vi "timing_channel_reference.get.vi"(8 "error in (no error)":errorcluster, 11 "Item Ref in":T1 format="%.0x") -> (0 "error out":errorcluster, 2 "Timing Channel Ref":T1=18446744073709551615 format="%.0x", 3 "Item Ref out":T1=18446744073709551615 format="%.0x")   [LabVIEW 2024, in "Nominal Client Scripting.lvlib"]
uses:
  <vilib>/NI VeriStand/Custom Device API/Custom Device Item Ref.ctl
  Nominal Client Scripting.lvlib
  <vilib>/NI VeriStand/Custom Device Tools/Custom Device Utility Library/Custom Device Utility Library.lvlib
  <vilib>/NI VeriStand/Custom Device API/Custom Device API.lvlib
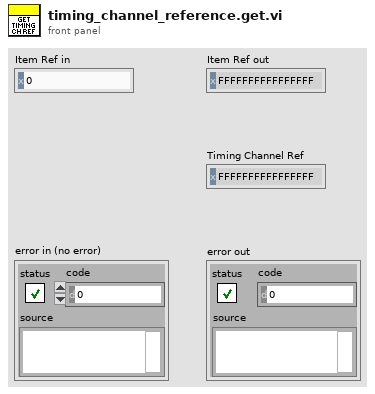
[diagram p1: front panel]
types:
  T1 = typedef "Custom Device API.lvlib/Custom Device Item Ref.ctl" = u64
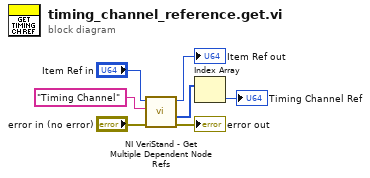
[diagram p0: block diagram]
diagram:
  n1 = call <vilib>:"NI VeriStand - Get Multiple Dependent Node Refs.vi"("error in (no error)"="error in (no error)", "Base Property Name"="Timing Channel" ("Property Name"), "Item Ref in"="Item Ref in") -> ("error out"=→"error out":errorcluster, "Dependent Node Refs"=w2:T1[], "Item Ref out"=→"Item Ref out":T1)  [unwired: 6 in]
  n2 = Index Array(array=w2) -> (element=→"Timing Channel Ref":T1)  [unwired: 1 in]
